vi "Square.vi"() -> ()   [LabVIEW 2012]
uses:
  <vilib>/Platform/TimedLoop/XDataNode/timing_clust.ctl
  <vilib>/Platform/TimedLoop/XDataNode/nitl_modes.ctl
  <vilib>/Platform/TimedLoop/XDataNode/wakeup.ctl
  <vilib>/Instr/_visa.llb/VISA Configure Serial Port (Instr).vi
  <vilib>/Platform/TimedLoop/XDataNode/XDataNode.xnode
  <vilib>/Platform/TimedLoop/XDataNode/XDNodeRunTimeDep.lvlib
panel:
  out "appended array":i32[](array[numeric])=[3, 1, 0, 1, 3, 1, 0, 1, 3, 1, 0, 1, 3, 1, 0, 1]
  in  "Turn Time":dbl=3.2
  in  "Fwd Time":i8=15
  out "error out":errorcluster
  in  "VISA resource name":refnum<visa-resource-name>="ASRL1::INSTR"
  out "Write Buffer":string="!B00\r"
  out "Write Error":bool
  out "Write Return Count":u32=5
  out "Read Error":bool
  out "Read Buffer":string="+\r"
  out "Current Step":i32=15
  out "Current Time":u32=406713
  out "Time Diff":u32=1050
  out "Last Time Inc":u32=406713
  out "x .or. y?":bool=TRUE
  out "Read Return Count":u32=2
  out "Read Buffer Log":string="+\r!B00\r+\r!B00\r+\r!B00\r+\r!B00\r+\r!B00\r+\r!B00\r+\r!B00\r+\r!B00\r+\r!B00\r+\r!B00\r+\r!B00\r+\r!B00\r+\r!B00\r+\r!B00\r+\r!B00\r+\r!B00\r+\r!B5F\r+\r!A00\r+\r!A00\r+\r!A00\r+\r!A00\r+\r!A00\r+\r!A00\r+\r!A00\r+\r!A00\r+\r!A00\r+\r!A00\r+\r!A00\r+\r!A00\r+\r!A00\r+\r!A00\r+\r!A00\r+\r!A00\r+\r!A00\r+\r!A00\r+\r!A00\r+\r!A00\r+\r!A00\r+\r!A32\r+\r!A32\r+\r!A32\r+\r!A32\r+\r!A32\r+\r!A32\r+\r!A32\r+\r!A32\r+\r!A32\r+\r!A32\r+\r!A32\r+\r!A32\r+\r!A32\r+\r!A32\r+\r!A32\r+\r!A32\r+\r!A32\r+\r!A32\r+\r!A32\r+\r!A32\r+\r!A32\r+\r!A32\r+\r!A32\r+\r!A32\r+\r!A32\r+\r!A32\r+\r!A32\r+\r!A32\r+\r!A32\r+\r!A32\r+\r!A32\r+\r!A32\r+\r!A32\r+\r!A32\r+\r!A32\r+\r!A32\r+\r!A32\r+\r!A32\r+\r!A32\r+\r!A32\r+\r!A32\r+\r!A32\r+\r!A32\r+\r!A32\r+\r!A32\r+\r!A32\r+\r!A32\r+\r!A32\r+\r!A32\r+\r!A32\r+\r!A32\r+\r!A32\r+\r!A32\r+\r!A32\r+\r!A32\r+\r!A32\r+\r!A32\r+\r!A32\r+\r!A32\r+\r!A32\r+\r!A32\r+\r!B00\r+\r!B00\r+\r!B00\r+\r!B00\r+\r!B00\r+\r!B00\r+\r!B00\r+\r!B00\r+\r!B00\r+\r!B00\r+\r!B00\r+\r!B00\r+\r!B00\r+\r!B00\r+\r!B00\r+\r!B00\r+\r!B00\r+\r!B00\r+\r!B00\r+\r!B00\r+\r!B00\r+\r!B5F\r+\r!A00\r+\r!A00\r+\r!A00\r+\r!A00\r+\r!A00\r+\r!A00\r+\r!A00\r+\r!A00\r+\r!A00\r+\r!A00\r+\r!A00\r+\r!A00\r+\r!A00\r+\r!A00\r+\r!A00\r+\r!A00\r+\r!A00\r+\r!A00\r+\r!A00\r+\r!A00\r+\r!A00\r+\r!A32\r+\r!A32\r+\r!A32\r+\r!A32\r+\r!A32\r+\r!A32\r+\r!A32\r+\r!A32\r+\r!A32\r+\r!A32\r+\r!A32\r+\r!A32\r+\r!A32\r+\r!A32\r+\r!A32\r+\r!A32\r+\r!A32\r+\r!A32\r+\r!A32\r+\r!A32\r+\r!A32\r+\r!A32\r+\r!A32\r+\r!A32\r+\r!A32\r+\r!A32\r+\r!A32\r+\r!A32\r+\r!A32\r+\r!A32\r+\r!A32\r+\r!A32\r+\r!A32\r+\r!A32\r+\r!A32\r+\r!A32\r+\r!A32\r+\r!A32\r+\r!A32\r+\r!A32\r+\r!A32\r+\r!A32\r+\r!A32\r+\r!A32\r+\r!A32\r+\r!A32\r+\r!A32\r+\r!A32\r+\r!A32\r+\r!A32\r+\r!A32\r+\r!A32\r+\r!A32\r+\r!A32\r+\r!A32\r+\r!A32\r+\r!A32\r+\r!A32\r+\r!A32\r+\r!A32\r+\r!A32\r\r\r\r\r\r\r\r\r\r\r"
  out "Start Time":u32=385935
  in  "Stop":bool
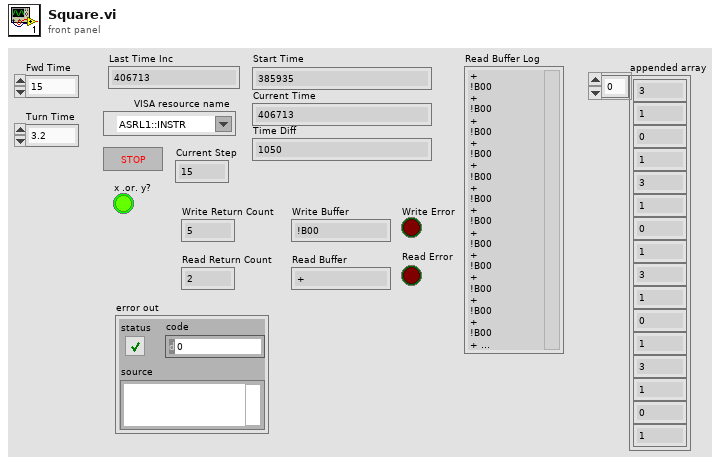
[diagram p1: front panel]
types:
  T1 = typedef "XDNodeRunTimeDep.lvlib/timing_clust.ctl" = cluster{"Expected End [f-1]":u64, "Actual End [f-1]":u64, "Finished Late? [f-1]":bool, "Expected End [i-1]":u64, "Actual End [i-1]":u64, "Finished Late? [i-1]":bool, "Expected Start [i]":u64, "Actual Start [i]":u64, "Expected Start [f]":u64, "Actual Start [f]":u64, "Source Name":string, "Structure Name":string, "Period":i64, "Deadline":i64, "Offset":i64, "Start":i64, "Priority":i32, "Timeout":i32, "Mode":T2, "Wakeup Reason":T3, "Error":errorcluster, "Source Type":string, "Secondary Source Type":string, "Global End Time":u64, "Global Start Time":u64, "Frame Duration":u64, "Iteration Duration":u64, "Assigned CPU":i32, "I/O Scan Engine Mode":u32}
  T2 = typedef "XDNodeRunTimeDep.lvlib/nitl_modes.ctl" = enum32{"No Change", "Process missed periods, maintain original phase", "Discard missed periods, maintain original phase", "Process missed periods, ignore original phase", "Discard missed periods, ignore original phase"}
  T3 = typedef "XDNodeRunTimeDep.lvlib/wakeup.ctl" = enum32{"Normal", "Aborted", "Asynchronous wakeup", "Timing source error", "Timed loop error", "Timeout"}
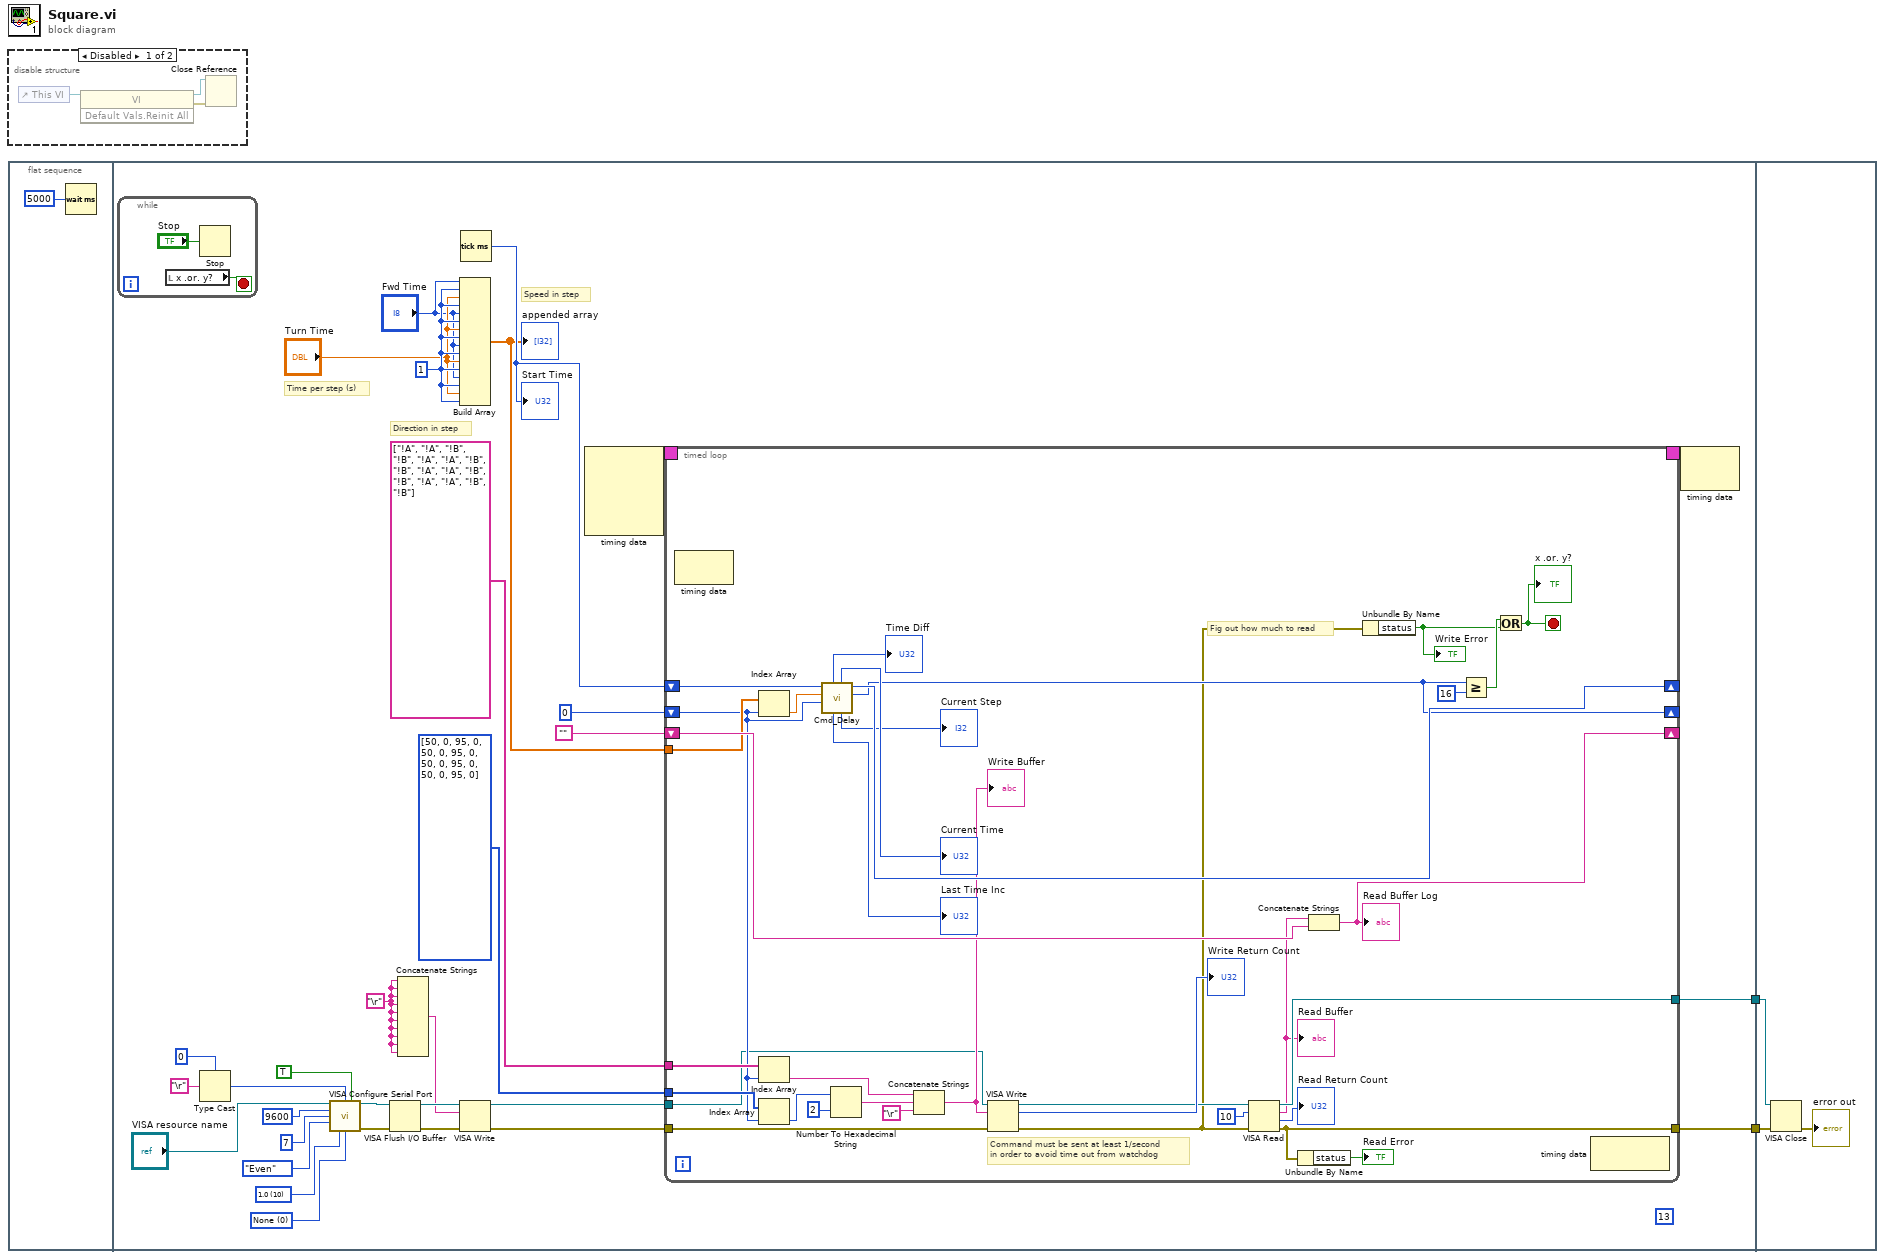
[diagram p0: block diagram]
diagram:
  n1 = disable-structure shown="Disabled" {
    frame Disabled {
      n2 = control-ref of="This VI"() -> (w5:refnum<vi>)
      n3 = invoke class="VI" method="Default Vals.Reinit All"(reference=w5) -> (reference out=w3:refnum<vi>, error out=w4:errorcluster)  [unwired: 2 in, 1 out]
      n4 = Close Reference(reference=w3, error in (no error)=w4) -> ()  [unwired: 1 out]
    }
    frame Enabled {
    }
  }
  n5 = flat-sequence {
    tunnel: [w33] -> w2
    tunnel: [w32] -> w1
    tunnel: w2 -> [w81]
    tunnel: w1 -> [w80]
    frame #0 {
      n6 = Wait (ms)(milliseconds to wait=u32 5000) -> ()  [unwired: 1 out]
    }
    frame #1 {
      w10 = 1
      w12 = "\r"
      (unwired) u8 13 ("termination char\n(0xA = '\\n' = LF)")
      w34 = u16 0 items=["None", "XON/XOFF", "RTS/CTS", "XON/XOFF & RTS/CTS", "DTR/DSR", "XON/XOFF & DTR/DSR"] ("flow control (0:none)")
      w35 = u16 10 items=["1.0"=10, "1.5"=15, "2.0"=20] ("stop bits (10: 1 bit)")
      # "Direction in step"
      # "Speed in step"
      # "Time per step (s)"
      n7 = while {
        stop <- w77 stop-if-true
        n8 = local read "x .or. y?"() -> (w77:bool)
        n9 = Stop(stop? (T)="Stop") -> ()
      }
      n10 = Type Cast(type=u8 0, x="\r") -> (*(type *) &x=w11:u8)
      n11 = call-poly "VISA Configure Serial Port"("VISA resource name"="VISA resource name", "termination char\n(0xA = '\\n' = LF)"=w11, "Enable Termination\nChar (T)"=TRUE ("Enable Termination\nChar (T)"), "baud rate (9600)"=u32 9600, "data bits (8)"=u16 7, "parity (0:none)"=enum16{"None", "Odd", "Even", "Mark", "Space"}."Even", "stop bits (10: 1 bit)"=w35, "flow control (0:none)"=w34) -> ("VISA resource name out"=w26:refnum<visa-resource-name>, "error out"=w25:errorcluster)  [unwired: 6 in]
      n12 = VISA Flush I/O Buffer(VISA resource name=w26, error in (no error)=w25) -> (VISA resource name out=w15:refnum<visa-resource-name>, error out=w14:errorcluster)  [unwired: 1 in]
      n13 = Concatenate Strings(w12, w12, w12, w12, w12, w12, w12, w12, w12, w12) -> (w13:string)
      n14 = Build Array("Fwd Time", w10, "Turn Time", w10, "Fwd Time", w10, "Turn Time", w10, "Fwd Time", w10, "Turn Time", w10, "Fwd Time", w10, "Turn Time", w10) -> (w7:dbl[])
      "appended array" <- w7
      n15 = VISA Write(VISA resource name=w15, write buffer=w13, error in (no error)=w14) -> (VISA resource name out=w16:refnum<visa-resource-name>, error out=w17:errorcluster)  [unwired: 1 out]
      n16 = Tick Count (ms)() -> (millisecond timer value=w27:u32)
      "Start Time" <- w27
      n17 = node-c288() -> (w19:T1)  [unwired: 4 in]
      n18 = timed-loop {
        tunnel: w16 -> [w39]
        tunnel: [w71] -> w33
        tunnel: [w70] -> w32
        tunnel: w17 -> [w38]
        shift-right: [w67] -> _
        shift-left: "" -> [w66]
        shift-right: [w50] -> _
        shift-left: u32 0 ("millisecond timer value") -> [w51]
        tunnel: string[] ["!A", "!A", "!B", "!B", "!A", "!A", "!B", "!B", "!A", "!A", "!B", "!B", "!A", "!A", "!B", "!B"] -> [w62]
        tunnel: i32[] [50, 0, 95, 0, 50, 0, 95, 0, 50, 0, 95, 0, 50, 0, 95, 0] -> [w61]
        tunnel: w7 -> [w60]
        shift-right: [w54] -> _
        shift-left: w27 -> [w58]
        timing: w19 -> [_]
        timing-out: [_] -> w18
        stop <- w40 stop-if-true
        # "Fig out how much to read"
        # "Command must be sent at least 1/second\nin order to avoid time out from watchdog"
        n19 = node-c288() -> ()  [unwired: 1 in, 1 out]
        n20 = Index Array(array=w60, index=w51) -> (element=w57:dbl)
        n21 = Index Array(array=w62, index=w51) -> (element=w59:string)
        n22 = Index Array(array=w61, index=w51) -> (element=w46:i32)
        n23 = call "Cmd_Delay.vi"("Cmd Number"=w51, "Cmd Duration"=w57, "Cmd Start Time In"=w58) -> ("Next Cmd Number"=w50:u32, "Cmd Start Time Out"=w54:u32, "Current Step"=→"Current Step":i32, "Current Time"=→"Current Time":u32, "Last Time Inc"=→"Last Time Inc":u32, "Time Diff"=→"Time Diff":u32)  [unwired: 3 in]
        n24 = Number To Hexadecimal String(1:i16 2 ("width (-)"), 2:w46) -> (0:w65:string)
        n25 = Concatenate Strings(w59, w65, "\r") -> (w47:string)
        "Write Buffer" <- w47
        n26 = VISA Write(VISA resource name=w39, write buffer=w47, error in (no error)=w38) -> (VISA resource name out=w44:refnum<visa-resource-name>, return count=→"Write Return Count":u32, error out=w43:errorcluster)
        n27 = VISA Read(VISA resource name=w44, byte count=u32 10, error in (no error)=w43) -> (VISA resource name out=w71:refnum<visa-resource-name>, read buffer=w64:string, return count=→"Read Return Count":u32, error out=w70:errorcluster)
        "Read Buffer" <- w64
        n28 = Unbundle By Name(w70) -> ("status"=→"Read Error":bool)
        n29 = Concatenate Strings(w64, w66) -> (w67:string)
        "Read Buffer Log" <- w67
        n30 = Unbundle By Name(w43) -> ("status"=w41:bool)
        "Write Error" <- w41
        n31 = Greater Or Equal?(x=w50, y=16) -> (x >= y?=w42:bool)
        n32 = Or(x=w42, y=w41) -> (x .or. y?=w40:bool)
        "x .or. y?" <- w40
        n33 = node-c288() -> ()  [unwired: 1 in, 1 out]
      }
      n34 = node-c288(w18) -> ()  [unwired: 1 out]
    }
    frame #2 {
      n35 = VISA Close(VISA resource name=w81, error in (no error)=w80) -> (error out=→"error out":errorcluster)
    }
  }
